vi "Tektronix 7000 Series Acquire Math Waveform.vi"() -> ()   [LabVIEW 2015]
doc: "Demonstrates how to use the Configure Math Expression (Unary Operation) VI and the Configure Math Expression (Binary Operation) VI. You can configure this VI to acquire math waveforms by following the following steps:\n\n1. Specify a valid VISA resource to use. \n2. Specify a math channel. \n3. Specify the operands of an expression.\n3. Specify a time-out value for reading a waveform.\n4. Run this VI. The <B>Waveform Graph</B> displays the waveform you acquire. \n\n<B>Note:</B> The TDS 5000 series will not support most unary functions or support nested functions without the math option installed. This restriction will cause this VI to return an error."
uses:
  <instrlib>/Tektronix 7000 Series/Public/Configure/Math/Configure Math Expression (Binary Operation).vi
  <instrlib>/Tektronix 7000 Series/Public/Configure/Math/Configure Math Expression (Unary Operation).vi
  <instrlib>/Tektronix 7000 Series/Public/Configure/Math/Configure Math (Advanced).vi
  <instrlib>/Tektronix 7000 Series/Public/Data/Read (Single Waveform).vi
  <instrlib>/Tektronix 7000 Series/Tektronix 7000 Series.lvlib
panel:
  in  "Maximum Time (10000 ms)":u32=10000
  in  "Operator (0: AVG)":u16(ring) items=["AVG", "SQRT", "FABS", "Integral", "Log10", "Ceil", "Derivative", "LogE", "Floor", "Invert", "Exp", "Sin", "Cos", "Tan", "ASin", "ACos", "ATan", "Sinh", "Cosh", "Tanh", "Min", "Max", "wfmDB", "Spectral Mag", "Spectral Real", "Spectral Phase", "Spectral Imaginary"]
  in  "Expression Input 2":string(combo)
  in  "Expression Input 1":string(combo)
  in  "Operator (0: Add)":u16(ring) items=["Add", "Subtract", "Multiply", "Divide"]
  in  "Destination (4:Math1)":u16(ring)=4 items=["Math 1"=4, "Math 2"=5, "Math 3"=6, "Math 4"=7]
  in  "VISA Resource Name":refnum<visa-resource-name>
  out "Waveform Graph":waveform(dbl)(graph)
  # "(c) 2006 - 2016 National Instruments Corporation.  ALL RIGHTS RESERVED."
  # "Math = Unary Operator( Binary Operator( Expression Input1, Expression Input2 ) )"
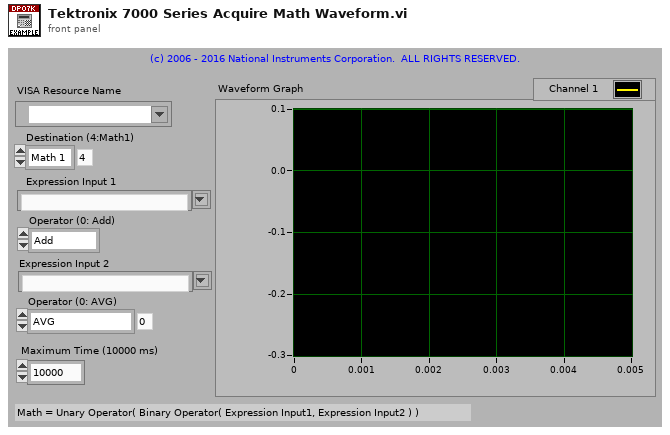
[diagram p1: front panel]
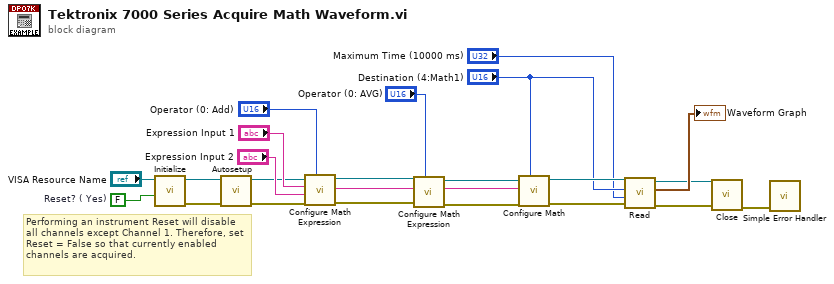
[diagram p0: block diagram]
diagram:
  w1 = FALSE  # Reset? ( Yes)
  # "Performing an instrument Reset will disable all channels except Channel 1. Therefore, set Reset = False so that currently enabled channels are acquired."
  n1 = call <instrlib>:"Initialize.vi"("Reset? ( Yes)"=w1, "VISA resource name"="VISA Resource Name") -> ("error out"=w4:errorcluster, "VISA resource name out"=w5:refnum<visa-resource-name>)  [unwired: 8 in]
  n2 = call <instrlib>:"Autosetup.vi"("error in (no error)"=w4, "VISA resource name"=w5) -> ("error out"=w2:errorcluster, "VISA resource name out"=w3:refnum<visa-resource-name>)  [unwired: 8 in]
  n3 = call-poly <instrlib>:"Configure Math Expression.vi"("Operator (0: Add)"="Operator (0: Add)", "error in (no error)"=w2, "Expression Input 2"="Expression Input 2", "Expression Input 1"="Expression Input 1", "VISA resource name"=w3) -> ("error out"=w11:errorcluster, "Expression Output"=w7:string, "VISA resource name out"=w12:refnum<visa-resource-name>)  [unwired: 4 in]
  n4 = call-poly <instrlib>:"Configure Math Expression.vi"("Operator (0: AVG)"="Operator (0: AVG)", "error in (no error)"=w11, "Expression Input 1"=w7, "VISA resource name"=w12) -> ("error out"=w9:errorcluster, "Expression Output"=w6:string, "VISA resource name out"=w10:refnum<visa-resource-name>)  [unwired: 5 in]
  n5 = call-poly <instrlib>:"Configure Math.vi"("Destination (4:Math1)"="Destination (4:Math1)", "error in (no error)"=w9, "Expression"=w6, "VISA resource name"=w10) -> ("error out"=w19:errorcluster, "VISA resource name out"=w20:refnum<visa-resource-name>)  [unwired: 6 in]
  n6 = call-poly <instrlib>:"Read.vi"("error in (no error)"=w19, "Maximum Time (10000 ms)"="Maximum Time (10000 ms)", "Channel (0: Channel 1)"="Destination (4:Math1)", "VISA resource name"=w20) -> ("error out"=w21:errorcluster, "Waveform Data"=→"Waveform Graph":waveform(dbl), "VISA resource name out"=w23:refnum<visa-resource-name>)  [unwired: 5 in]
  n7 = call <instrlib>:"Close.vi"("error in (no error)"=w21, "VISA resource name"=w23) -> ("error out"=w22:errorcluster)  [unwired: 9 in]
  n8 = call <vilib>:"Simple Error Handler.vi"("error in (no error)"=w22) -> ()  [unwired: 4 in, 5 out]
